vi "ActBalance.vi"(10 "MaxSpeed (ft/s)":dbl) -> (1 "XSpeedDemand":dbl, 3 "Done":bool)   [LabVIEW 2020]
doc: "Robot begins balancing towards the \"GyroZero\" position. \n\nInputs:\n-- MaxSpeed -- Double -- in ft/s, the MaxSpeed the robot can go (Has no effect above 1.5)\n\n\nOutputs:\n-- Done -- Bool -- has the robot reached its target distance\n-- LeftSpeedDemand -- Double -- Speed Demand for left drive train inorder to reach target -- \n-- RightSpeedDemand -- Double -- Speed Demand for left drive train inorder to reach target --"
uses:
  <vilib>/Rock Robotics/WPI/ThirdParty/JAS_Junk/TrajLib/VI/Util_GetTime_U32.vi
  <vilib>/Rock Robotics/WPI/ThirdParty/JAS_Junk/TrajLib/LinearFilter_ResetToValue.vi
  <vilib>/Rock Robotics/WPI/ThirdParty/JAS_Junk/TrajLib/LinearFilter_Calculate.vi
  <vilib>/Rock Robotics/WPI/ThirdParty/JAS_Junk/TrajLib/Timer_New.vi
  <vilib>/Rock Robotics/SystemInterfaces/Utilities/FPGA_UtilitiesRead LocalTime.vi
  <vilib>/Rock Robotics/WPI/ThirdParty/JAS_Junk/TrajLib/VI/Util_GetTime_U64.vi
  <vilib>/Rock Robotics/Network Tables/NT Write Number.vi
  <vilib>/Rock Robotics/WPI/ThirdParty/JAS_Junk/TrajLib/LinearFilter_MovingAverage.vi
  <vilib>/Rock Robotics/WPI/ThirdParty/JAS_Junk/TrajLib/LinearFilter_LowPassBW1.vi
  <vilib>/Rock Robotics/WPI/ThirdParty/JAS_Junk/TrajLib/LinearFilter_LowPassBW2.vi
  <vilib>/Rock Robotics/WPI/ThirdParty/JAS_Junk/TrajLib/LinearFilter_HighPassBW1.vi
  <vilib>/Rock Robotics/WPI/ThirdParty/JAS_Junk/TrajLib/LinearFilter_HighPassBW2.vi
  <vilib>/Utility/semaphor.llb/Obtain Semaphore Reference.vi
  <vilib>/Rock Robotics/WPI/ThirdParty/JAS_Junk/TrajLib/Timer_Reset.vi
  <vilib>/Rock Robotics/WPI/ThirdParty/JAS_Junk/TrajLib/Timer_Start.vi
  <vilib>/Rock Robotics/WPI/ThirdParty/JAS_Junk/TrajLib/Timer_HasPeriodPassedOnce.vi
  <vilib>/Rock Robotics/WPI/ThirdParty/JAS_Junk/TrajLib/Timer_Stop.vi
  <vilib>/Rock Robotics/WPI/ThirdParty/JAS_Junk/TrajLib/Trajectory_Library.lvlib
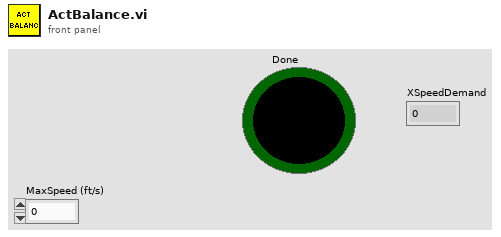
[diagram p1: front panel]
types:
  T1 = enum16{"Moving Average", "Low Pass 1st Order Butterworth", "Low Pass 2nd Order Butterworth", "High Pass 1st Order Butterworth", "High Pass 2nd Order Butterworth"}
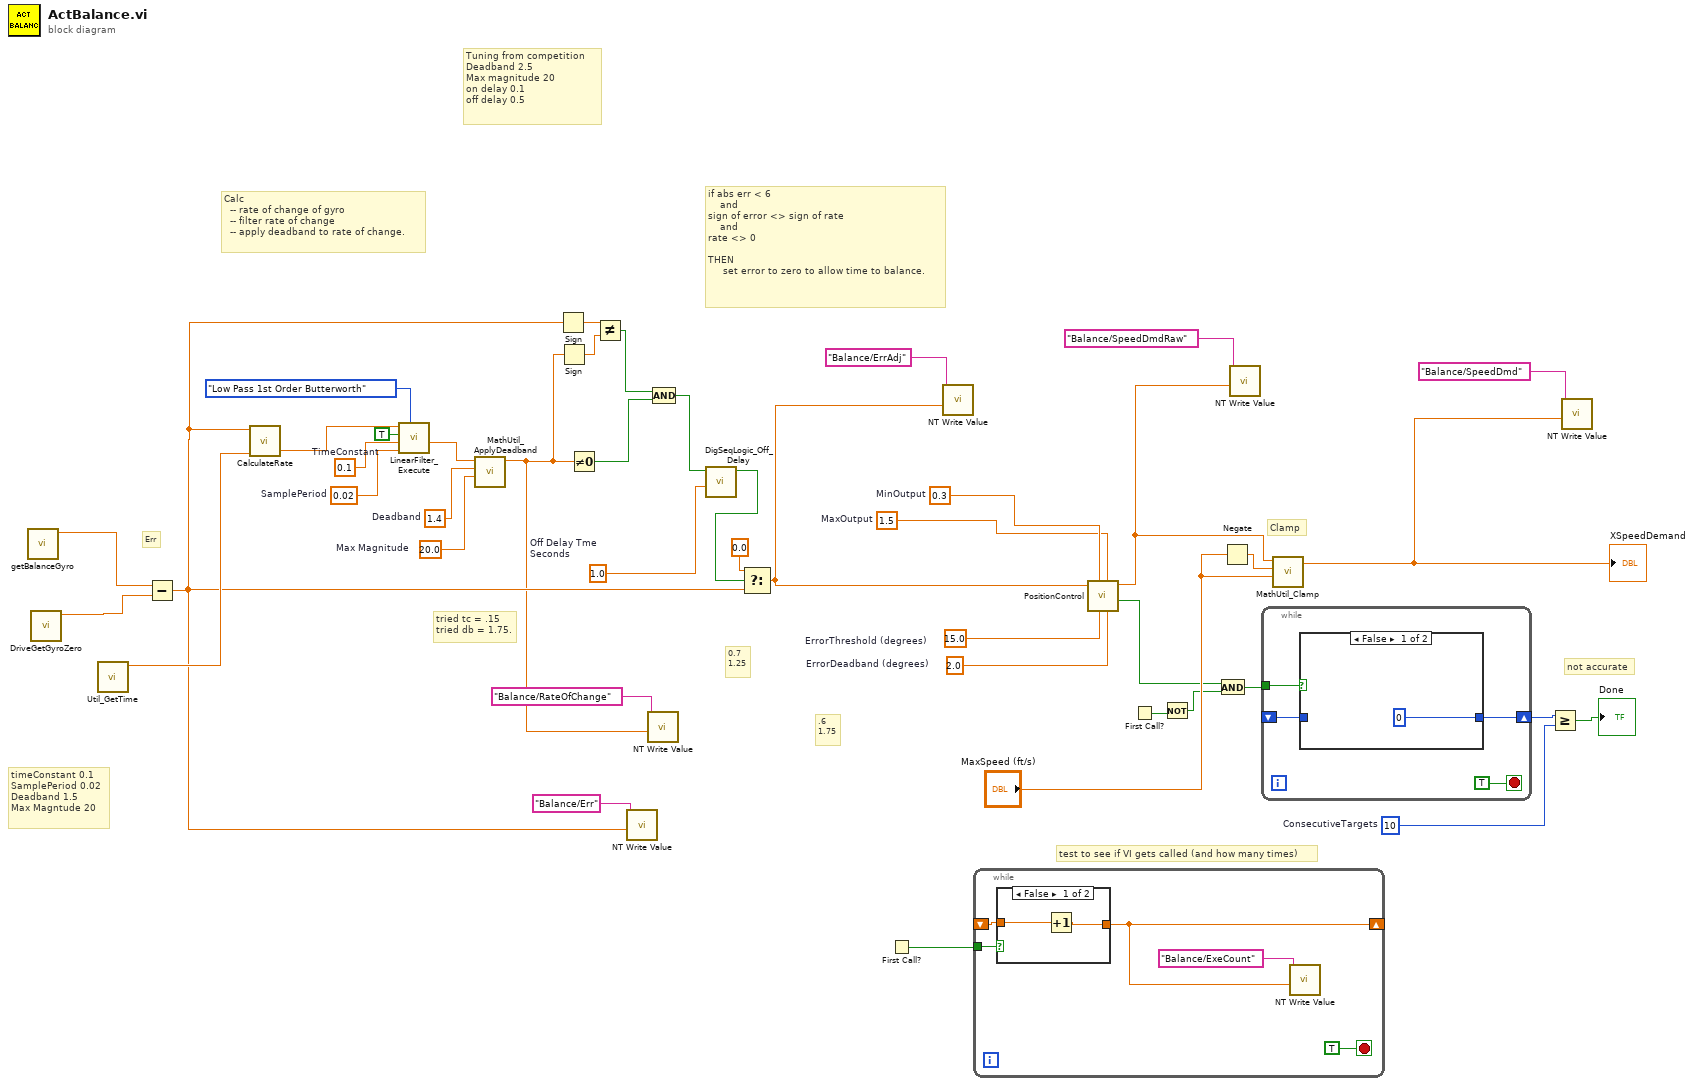
[diagram p0: block diagram]
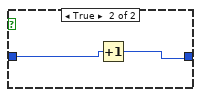
[diagram p2: hidden frame]
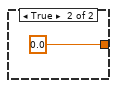
[diagram p3: hidden frame]
diagram:
  w16 = 1.0  # Off Delay Tme Seconds
  w34 = 0.02  # SamplePeriod
  w33 = 0.1  # TimeConstant
  w35 = 20.0  # Max Magnitude
  w36 = 1.4  # Deadband
  w12 = 1.5  # MaxOutput
  w13 = 0.3  # MinOutput
  w8 = 10  # ConsecutiveTargets
  w10 = 2.0  # ErrorDeadband (degrees)
  w11 = 15.0  # ErrorThreshold (degrees)
  # "Tuning from competition\nDeadband 2.5\nMax magnitude 20\non delay 0.1\noff delay 0.5"
  # ".6\n1.75"
  # "test to see if VI gets called (and how many times)"
  # "not accurate"
  # "if abs err < 6 \n    and\nsign of error <> sign of rate\n    and\nrate <> 0\n\nTHEN\n     set error to zero to allow time to balance."
  # "tried tc = .15\ntried db = 1.75."
  # "Calc\n  -- rate of change of gyro\n  -- filter rate of change\n  -- apply deadband to rate of change."
  # "Err"
  # "0.7\n1.25"
  # "timeConstant 0.1\nSamplePeriod 0.02\nDeadband 1.5\nMax Magntude 20"
  # "Clamp"
  n1 = call "getBalanceGyro.vi"() -> ("BalanceGyroReading"=w2:dbl)  [unwired: 11 in]
  n2 = call "DriveGetGyroZero.vi"() -> ("GyroZero"=w1:dbl)  [unwired: 11 in]
  n3 = call <vilib>:"Util_GetTime.vi"() -> ("FPGA_Time_Seconds"=w37:dbl)  [unwired: 9 in, 2 out]
  n4 = Subtract(x=w2, y=w1) -> (x-y=w26:dbl)
  n5 = call "CalculateRate.vi"("Time (s)"=w37, "Distance (units)"=w26) -> ("Rate (units/s)"=w29:dbl)  [unwired: 9 in]
  n6 = call <vilib>:"LinearFilter_Execute.vi"("Filter Type"=T1."Low Pass 1st Order Butterworth", "SamplePeriod"=w34, "TimeConstant"=w33, "Enable"=TRUE, "Input"=w29) -> ("Output"=w28:dbl)  [unwired: 5 in, 1 out]
  n7 = call <vilib>:"MathUtil_ApplyDeadband.vi"("Max Magnitude"=w35, "Deadband"=w36, "Value"=w28) -> ("Result"=w17:dbl)  [unwired: 8 in]
  n8 = Sign(1:w26) -> (0:w40:dbl)
  n9 = Sign(1:w17) -> (0:w39:dbl)
  n10 = Not Equal To 0?(x=w17) -> (x != 0?=w30:bool)
  n11 = Not Equal?(x=w40, y=w39) -> (x != y?=w38:bool)
  n12 = call-poly <vilib>:"NT Write Value.vi"("value"=w26, "name"="Balance/Err") -> ()  [unwired: 9 in, 1 out]
  n13 = call-poly <vilib>:"NT Write Value.vi"("value"=w17, "name"="Balance/RateOfChange") -> ()  [unwired: 9 in, 1 out]
  n14 = Compound Arithmetic op=AND(w38, w30) -> (w14:bool)
  n15 = call <vilib>:"DigSeqLogic_Off_Delay.vi"("Delay"=w16, "Input"=w14) -> ("Output"=w15:bool)  [unwired: 8 in, 1 out]
  n16 = Select(t=0.0, s=w15, f=w26) -> (s? t:f=w24:dbl)
  n17 = First Call?() -> (First Call?: T/F=w19:bool)
  n18 = call-poly <vilib>:"NT Write Value.vi"("value"=w24, "name"="Balance/ErrAdj") -> ()  [unwired: 9 in, 1 out]
  n19 = while {
    tunnel: w19 -> [w47]
    shift-right: [w44] -> _
    shift-left: _ -> [w46]
    stop <- TRUE stop-if-true
    n20 = case shown="False" w47 {
      tunnel: [w50 0.0] -> w44
      tunnel: w46 -> [w49 _]
      frame False {
        n21 = Increment(x=w49) -> (x+1=w50:dbl)
      }
      frame True {
      }
    }
    n22 = call-poly <vilib>:"NT Write Value.vi"("value"=w44, "name"="Balance/ExeCount") -> ()  [unwired: 9 in, 1 out]
  }
  n23 = call "PositionControl.vi"("deadband"=w10, "maxdemand"=w12, "threshold"=w11, "mindemand"=w13, "Error"=w24) -> ("on target"=w3:bool, "output variable"=w22:dbl)  [unwired: 5 in]
  n24 = First Call?() -> (First Call?: T/F=w6:bool)
  n25 = Not(x=w6) -> (.not. x?=w4:bool)
  n26 = And(x=w3, y=w4) -> (x .and. y?=w5:bool)
  n27 = Negate(x="MaxSpeed (ft/s)") -> (-x=w43:dbl)
  n28 = call-poly <vilib>:"NT Write Value.vi"("value"=w22, "name"="Balance/SpeedDmdRaw") -> ()  [unwired: 9 in, 1 out]
  n29 = while {
    tunnel: w5 -> [w54]
    shift-right: [w53] -> w9
    shift-left: _ -> [w52]
    stop <- TRUE stop-if-true
    n30 = case shown="False" w54 {
      tunnel: [0 w57] -> w53
      tunnel: w52 -> [_ w58]
      frame False {
      }
      frame True {
        n31 = Increment(x=w58) -> (x+1=w57:i32)
      }
    }
  }
  n32 = call <vilib>:"MathUtil_Clamp.vi"("High Limit"="MaxSpeed (ft/s)", "Low Limit"=w43, "Value"=w22) -> ("Result"=w20:dbl)  [unwired: 8 in]
  "XSpeedDemand" <- w20
  n33 = Greater Or Equal?(x=w9, y=w8) -> (x >= y?=→"Done":bool)
  n34 = call-poly <vilib>:"NT Write Value.vi"("value"=w20, "name"="Balance/SpeedDmd") -> ()  [unwired: 9 in, 1 out]
